vi "相机1图像处理.vi"(9 "自动":bool, 10 "生产统计1":T3 {"良率" format="%#.2g"}, 11 "Img输入":T2) -> (0 "良率统计out":T3 {"良率" format="%#.2g"}, 1 "1处理时间":u16, 2 "1结果":bool=TRUE, 3 "Img输出":T2(plugin-control))   [LabVIEW 2014]
uses:
  Global.vi
  Controls/ProductNum.ctl
  <vilib>/vision/Image Controls.llb/IMAQ Image.ctl
panel:
  out "存档数据":T1
  out "方向正(针尖超下)?":bool
  out "数组":dbl[](array[numeric])
  in  "显示坐标":cluster{dbl, "Numeric":dbl}[](array[cluster])=[{300.0, "Numeric"=200.0}, {300.0, "Numeric"=300.0}, {300.0, "Numeric"=400.0}, {300.0, "Numeric"=500.0}, {300.0, "Numeric"=600.0}, {300.0, "Numeric"=700.0}, {300.0, "Numeric"=800.0}]
  in  "Img Path":path
  # "%"
  # "%"
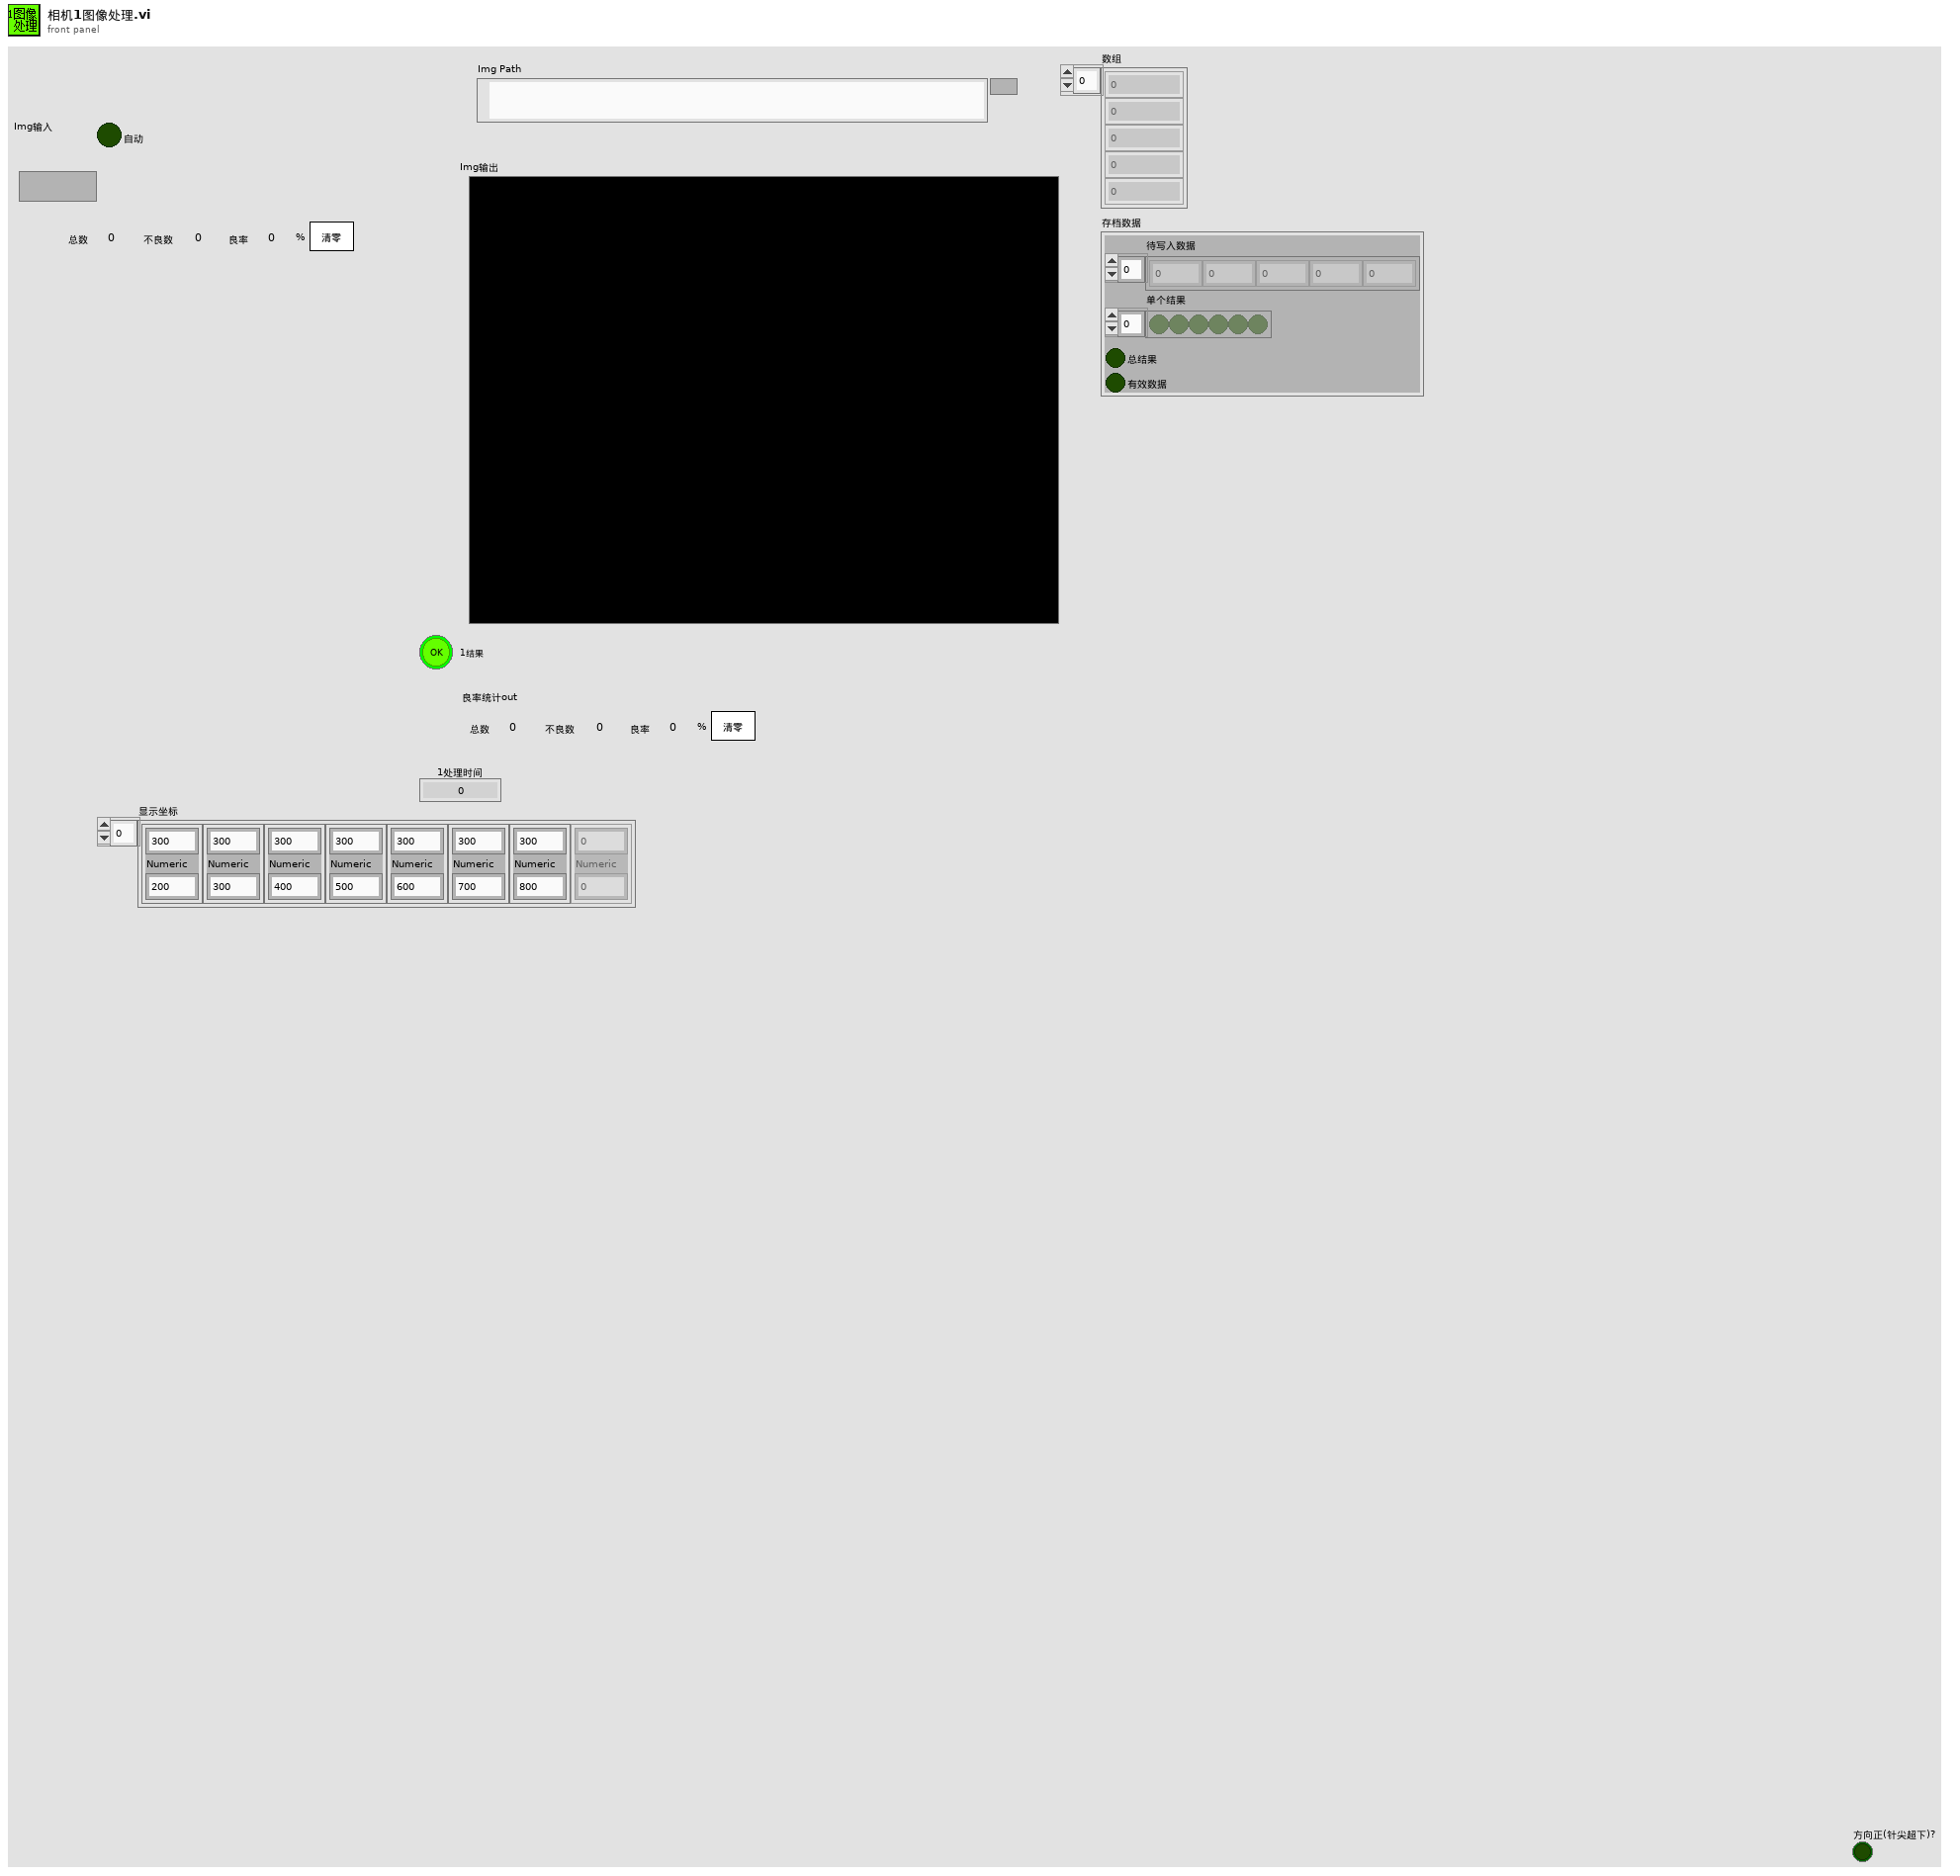
[diagram p1: front panel]
types:
  T1 = typedef "控件-存档数据和结果.ctl" = cluster{"待写入数据":dbl[], "单个结果":bool[], "总结果":bool, "有效数据":bool}
  T2 = typedef "IMAQ Image.ctl" = refnum<image>
  T3 = typedef "ProductNum.ctl" = cluster{"总数":u64, "不良数":u64, "良率":dbl, "清零":bool}
  T4 = typedef "ModeEditeControl.ctl" = cluster{"AllModelFold":path, "AllModelNamePath":path, "所有零件型号":string[], "当前零件型号":string, "所有建立零件信息":string[][], "当前零件序号":i32, "当前产品信息":T5}
  T5 = typedef "ModelInfo.ctl" = cluster{"产品型号":string, "二维码拍照":u32, "Mark点拍照":u32}
  T6 = cluster{"Desired Font (Application)":enum16{"User-specified Font", "Application Font", "System Font", "Dialog Font"}, "[User-specified Font]":cluster{"Font Name":string, "Size":i16, "Strikeout?":bool, "Italic?":bool, "Underline?":bool, "Outline?":bool, "Shadow?":bool, "Bold?":bool, "Rotation Angle":dbl}, "Horizontal Alignment":i16, "Vertical Alignment":i16}
  T7 = typedef "升立德IOAction.ctl" = enum16{"IO卡初始化", "读信号(16bit)", "写信号(16bit)", "写拍照Mark1完成信号OFF", "写拍照Mark1完成信号ON", "写拍照Mark2完成信号OFF", "写拍照Mark2完成信号ON", "写拍照Mark失败", "写拍照二维码完成信号ON", "写拍照二维码完成信号OFF", "GetInfo", "清除目标"}
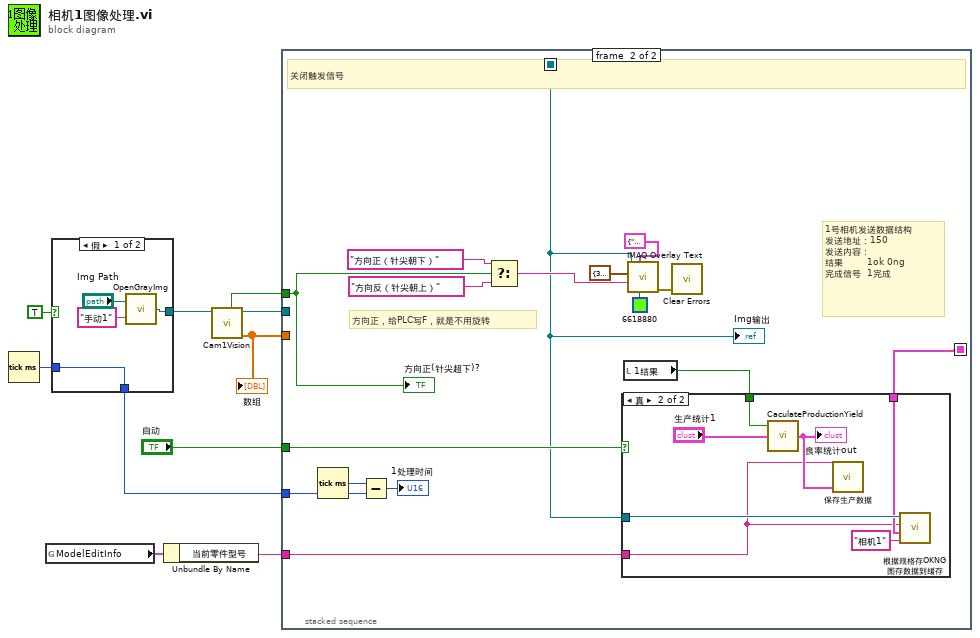
[diagram p0: block diagram]
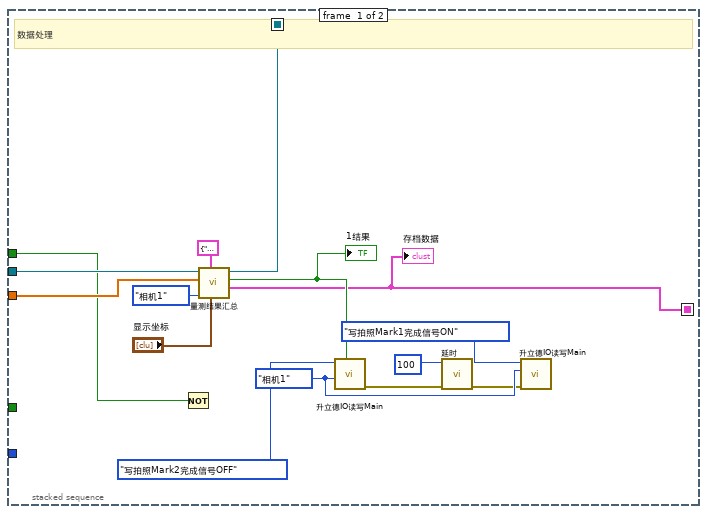
[diagram p2: hidden frame]
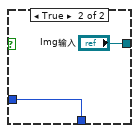
[diagram p4: hidden frame]
diagram:
  n1 = Tick Count (ms)() -> (millisecond timer value=w2:u32)
  n2 = global read "Global.vi" "ModelEditInfo"() -> (w7:T4)
  n3 = case shown="假" TRUE {
    tunnel: [w14 "Img输入"] -> w6
    tunnel: [w11 w15] -> w3
    tunnel: w2 -> [w11 w15]
    frame False {
      n4 = call "OpenGrayImg.vi"("Image Name"="手动1", "Img Path"="Img Path") -> ("Image Out"=w14:T2)
    }
    frame True {
    }
  }
  n5 = Unbundle By Name(w7) -> ("当前零件型号"=w4:string)
  n6 = call "Cam1Vision.vi"("Image in"=w6) -> ("方向正?针尖在右"=w1:bool, "Image Out"=w5:T2, "数组"=w8:dbl[])  [unwired: 5 in, 1 out]
  "数组" <- w8
  n7 = stacked-sequence {
    seq-local: [w26 _] -> [_ w32]
    seq-local: [w24 _] -> [_ w42]
    tunnel: w3 -> [_ w46]
    tunnel: "自动" -> [_ w43]
    tunnel: w8 -> [w27 _]
    tunnel: w5 -> [w28 _]
    tunnel: w4 -> [_ w41]
    tunnel: w1 -> [w18 w33]
    frame #0 {
      w29 = enum16{"相机1", "相机2", "相机3", "相机4"}."相机1" ("选择相机")
      # "数据处理"
      n8 = Not(x=w18) -> ()  [unwired: 1 out]
      n9 = call "量测结果汇总.vi"("显示坐标"="显示坐标", "Font, Size & Style"=T6 {"Desired Font (Application)"=enum."User-specified Font", "[User-specified Font]"={"Font Name"="", "Size"=80, "Strikeout?"=FALSE, "Italic?"=FALSE, "Underline?"=FALSE, "Outline?"=FALSE, "Shadow?"=FALSE, "Bold?"=FALSE, "Rotation Angle"=0.0}, "Horizontal Alignment"=0, "Vertical Alignment"=0}, "选项"=enum16{"相机1", "相机2", "相机3", "相机4"}."相机1", "量测数据1维"=w27, "Img in"=w28) -> ("存档数据"=w24:T1, "结果"=w25:bool, "ImgOut"=w26:T2)  [unwired: 2 in]
      "1结果" <- w25
      "存档数据" <- w24
      n10 = call "升立德IO读写Main.vi"(7:w25, "选择相机"=w29, "选项"=升立德IOAction."写拍照Mark2完成信号OFF") -> ("error out"=w20:errorcluster)  [unwired: 4 in, 4 out]
      n11 = call "延时.vi"("错误in"=w20, "等待时间（毫秒）"=u32 100) -> ("错误in"=w19:errorcluster)  [unwired: 9 in]
      n12 = call "升立德IO读写Main.vi"("error in"=w19, "选择相机"=w29, "选项"=升立德IOAction."写拍照Mark1完成信号ON") -> ()  [unwired: 4 in, 5 out]
    }
    frame #1 {
      # "方向正，给PLC写F，就是不用旋转"
      # "1号相机发送数据结构\n发送地址：150\n发送内容：\n结果        1ok 0ng\n完成信号  1完成"
      # "关闭触发信号"
      n13 = Tick Count (ms)() -> (millisecond timer value=w45:u32)
      n14 = Subtract(x=w45, y=w46) -> (x-y=→"1处理时间":u32)
      n15 = Select(t="方向正（针尖朝下）", s=w33, f="方向反（针尖朝上）") -> (s? t:f=w36:string)
      n16 = local read "1结果"() -> (w44:bool)
      n17 = case shown="真" w43 {
        tunnel: w44 -> [_ w53]
        tunnel: w32 -> [_ w51]
        tunnel: w42 -> [_ w49]
        tunnel: w41 -> [_ w48]
        frame False {
        }
        frame True {
          n18 = call "CaculateProductionYield.vi"("生产统计"="生产统计1", "Result(in)"=w53) -> ("良率统计out"=w52:T3)  [unwired: 1 in]
          "良率统计out" <- w52
          n19 = call "保存生产数据.vi"("error out"=w52, "输入簇"=w48) -> ()  [unwired: 1 in]
          n20 = call "根据规格存OKNG图存数据到缓存.vi"("选择相机字符串"="相机1", "存档数据和结果"=w49, "当前零件型号"=w48, "Img输入"=w51) -> ()  [unwired: 8 in]
        }
      }
      n21 = call "IMAQ Overlay Text"("Text Color (black)"=u32 6618880, "Font, Size & Style"=T6 {"Desired Font (Application)"=enum."User-specified Font", "[User-specified Font]"={"Font Name"="", "Size"=80, "Strikeout?"=FALSE, "Italic?"=FALSE, "Underline?"=FALSE, "Outline?"=FALSE, "Shadow?"=FALSE, "Bold?"=TRUE, "Rotation Angle"=0.0}, "Horizontal Alignment"=0, "Vertical Alignment"=0}, "String"=w36, "Origin"=cluster{"X":i32, "Y":i32} {"X"=300, "Y"=100}, "Image"=w32) -> ("error out"=w35:errorcluster)  [unwired: 5 in, 1 out]
      n22 = call <vilib>:"Clear Errors.vi"("error in (no error)"=w35) -> ()  [unwired: 5 in, 2 out]
      "方向正(针尖超下)?" <- w33
      "Img输出" <- w32
    }
  }
